vi "Parse updateNewChat.vi"(8 "error in (no error)":errorcluster, 11 "JSON (UTF-8) String":string) -> (0 "error out":errorcluster, 2 "Telegram State":T1, 3 "Variant":variant)   [LabVIEW 2015, in "JSON Library.lvlib"]
doc: "Created IvanLis by LabVIEW Portal\nProfile: http://labviewportal.org/memberlist.php?mode=viewprofile&u=987\neMail: IvanLisanov@gMail.com\nTelegram: https://t.me/IvanLis"
uses:
  JSON Library.lvlib
  Telegram Library/TypeDef/Telegram State.ctl
  TypeDef/Chat.ctl
  Telegram Library/Telegram Library.lvlib
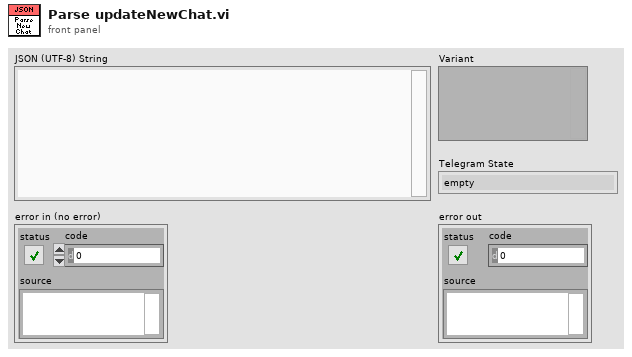
[diagram p1: front panel]
types:
  T1 = typedef "Telegram Library.lvlib/Telegram State.ctl" = enum16{"empty", "ok", "authorizationStateClosed", "authorizationStateWaitTdlibParameters", "authorizationStateWaitEncryptionKey", "authorizationStateWaitPhoneNumber", "authorizationStateWaitCode", "connectionStateWaitingForNetwork", "connectionStateConnectingToProxy", "connectionStateUpdating", "connectionStateConnecting", "connectionStateReady", "updateUser_user", "updateNewChat_chat", "updateNewMessage_Text", "updateChatLastMessage_Text", "updateDeleteMessages", "updateChatPosition", "ChatHistoryMessages_Text"}
  T2 = typedef "JSON Library.lvlib/Chat.ctl" = cluster{"@type":string, "id":i64, "title":string}
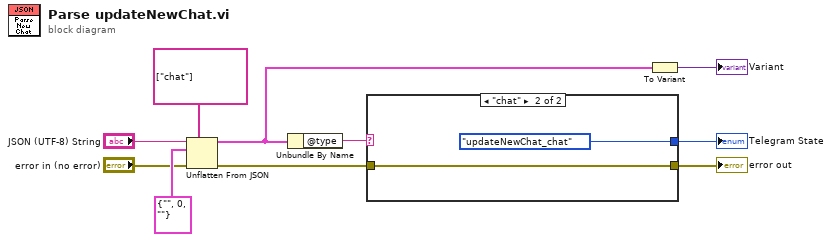
[diagram p0: block diagram]
diagram:
  n1 = Unflatten From JSON(path=string[] ["chat"], JSON string="JSON (UTF-8) String", type and defaults=T2 {"@type"="", "id"=0, "title"=""} ("value"), error in (no error)="error in (no error)") -> (value=w8:T2, error out=w7:errorcluster)  [unwired: 3 in]
  n2 = Unbundle By Name(w8) -> ("@type"=w6:string)
  n3 = case shown="\"chat\"" w6 {
    tunnel: w7 -> [w11 w13]
    tunnel: [w11 w13] -> w1
    tunnel: [_ Telegram_State."updateNewChat_chat" ("Telegram State")] -> w2
    frame Default {
    }
    frame "chat" {
    }
  }
  "Telegram State" <- w2
  "error out" <- w1
  n4 = To Variant(anything=w8) -> (Variant=→"Variant":variant)
